vi "JSONPacket Parse JSON.vi"(8 "error in (no error)":errorcluster, 10 "JSON String":string, 11 "JSONPacket in":refnum<class "JSONPacket.lvclass">) -> (0 "error out":errorcluster, 3 "JSONPacket out":refnum<class "JSONPacket.lvclass">)   [LabVIEW 2019, in "JSONPacket.lvclass"]
uses:
  JSONPacket.lvclass
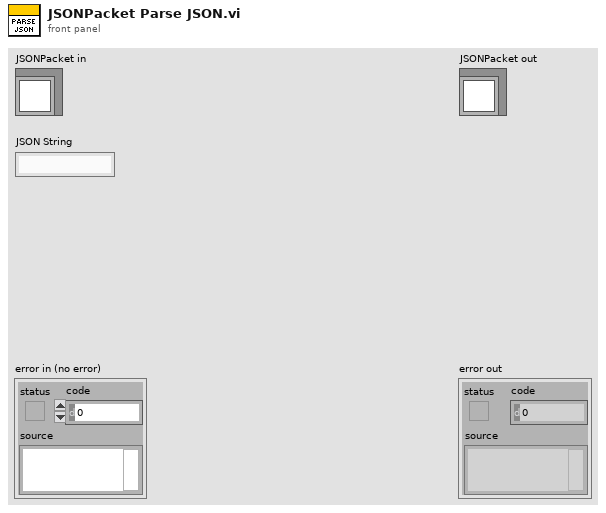
[diagram p1: front panel]
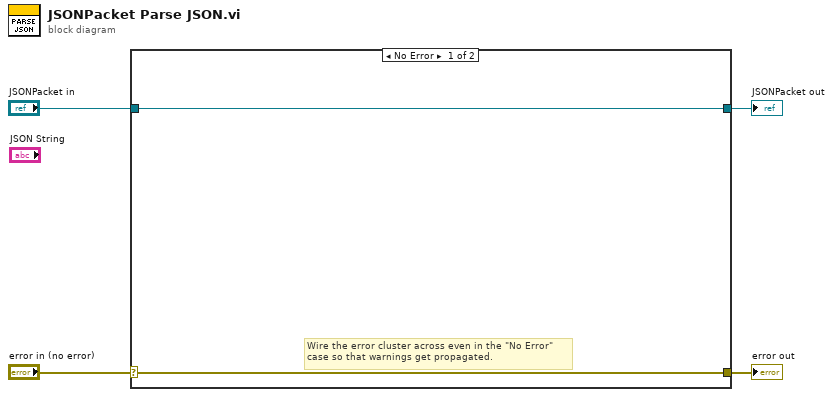
[diagram p0: block diagram]
diagram:
  n1 = case shown="No Error" "error in (no error)" {
    selector: "error in (no error)" -> [w5 w8]
    tunnel: [w5 w8] -> w3
    tunnel: [w6 w7] -> w1
    tunnel: "JSONPacket in" -> [w6 w7]
    frame No Error {
      # "Wire the error cluster across even in the \"No Error\"\ncase so that warnings get propagated."
    }
    frame Error {
    }
  }
  "error out" <- w3
  "JSONPacket out" <- w1
